vi "UT_006_LV to TOML.vi"() -> ()   [LabVIEW 2017]
uses:
  4ff207aa-191a-44af-8f7a-4e6e6b751422.vi
  <vilib>/addons/_JKI Toolkits/Caraya/classes/Assert/Assert True.vi
  lib/TOML to LabVIEW.vi
  <vilib>/addons/_JKI Toolkits/Caraya/classes/Assert/Assert Almost Equal_Float.vi
  <vilib>/addons/_JKI Toolkits/Caraya/classes/Test/Test.lvclass
  lib/TOML.lvlib
  <vilib>/addons/_JKI Toolkits/Caraya/classes/Assert/Assert.lvclass
panel:
  out "Cluster 2":T1={"2d-array-string"=[["a", "b", "c"], ["d", "e", "f"], ["g", "h", "i"]], "1d-array-float"=[3.14, nan, 1.123], "sub-cluster"={"string"="hello world", "path"=path "C:/dev/GitHub/.gitignore"}, "timestamp"=timestamp(3701448577.464638 s since 1904-01-01), "1d-array-cluster"=[{"string"="one", "int"=1}, {"string"="five", "int"=5}]}
  out "error out 2":errorcluster
  out "String":string
  in  "Cluster":T1={"2d-array-string"=[["a", "b", "c"], ["d", "e", "f"], ["g", "h", "i"]], "1d-array-float"=[3.14, nan, 1.123], "sub-cluster"={"string"="hello world", "path"=path "C:/dev/GitHub/.gitignore"}, "timestamp"=timestamp(3701448577.47 s since 1904-01-01), "1d-array-cluster"=[{"string"="one", "int"=1}, {"string"="five", "int"=5}]}
  out "error out":errorcluster
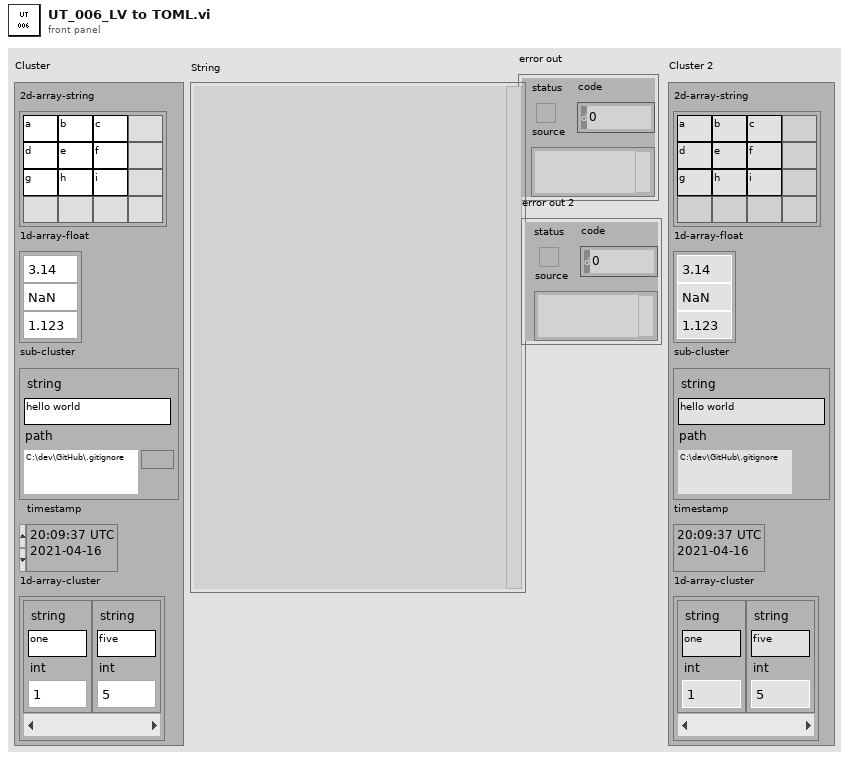
[diagram p1: front panel]
types:
  T1 = cluster{"2d-array-string":string[][], "1d-array-float":dbl[], "sub-cluster":cluster{"string":string, "path":path}, "timestamp":timestamp, "1d-array-cluster":cluster{"string":string, "int":i32}[]}
  T2 = typedef "TOML.lvlib/TOML Value.ctl" = cluster{"type":enum16{"Table", "Array", "String", "Integer", "Float", "Boolean", "Offset Date-Time", "Local Date-Time", "Local Date", "Local Time", "Path"}, "value":variant}
  T3 = cluster{"2d-array-string":bool[][], "1d-array-float":bool[], "sub-cluster":cluster{"string":bool, "path":bool}, "timestamp":bool, "1d-array-cluster":cluster{"string":bool, "int":bool}[]}
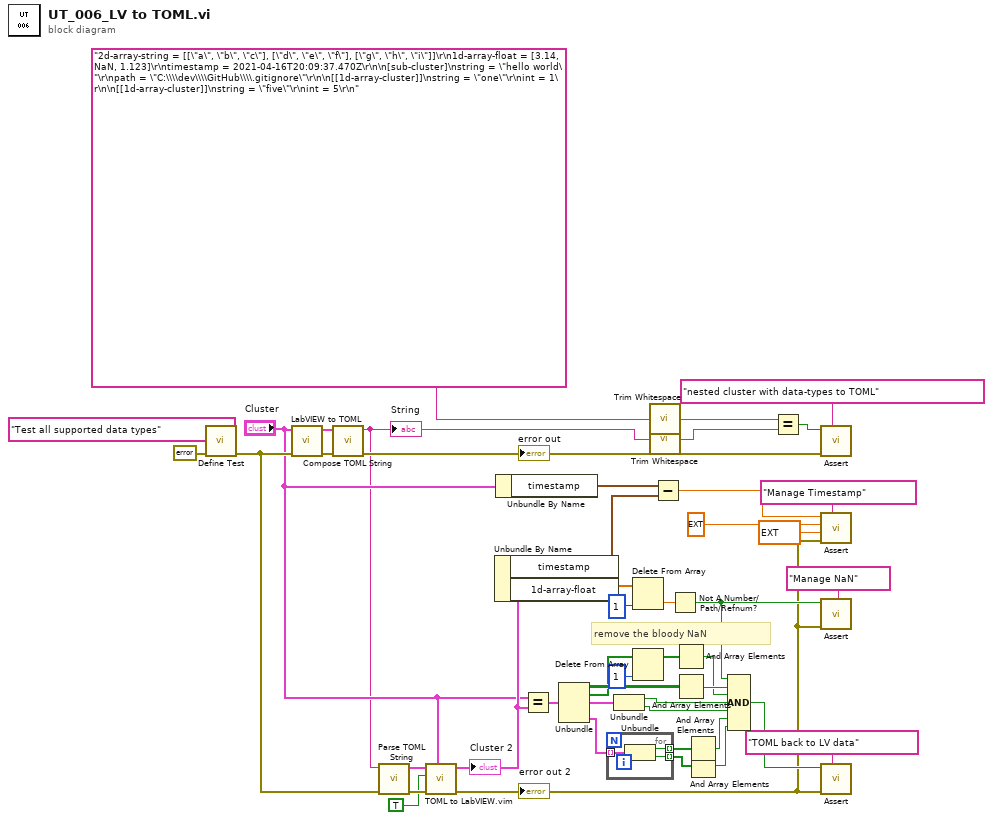
[diagram p0: block diagram]
diagram:
  # "remove the bloody NaN"
  n1 = call <vilib>:"Define Test.vi"("error in (no error)"=errorcluster {"status"=FALSE, "code"=0, "source"=""}, "Label (VI Title)"="Test all supported data types") -> ("error out"=w37:errorcluster)  [unwired: 9 in]
  n2 = call "LabVIEW to TOML.vi"("error in (no error)"=w37, "LV Value"="Cluster") -> ("error out"=w43:errorcluster, "TOML Value"=w36:T2)  [unwired: 7 in, 1 out]
  n3 = call "Compose TOML String.vi"("error in (no error)"=w43, "Value"=w36) -> ("error out"=w42:errorcluster, "String"=w2:string)  [unwired: 8 in]
  "error out" <- w42
  "String" <- w2
  n4 = call "Parse TOML String.vi"("error in (no error)"=w37, "String"=w2) -> ("error out"=w40:errorcluster, "Value"=w35:T2)  [unwired: 8 in]
  n5 = call "TOML to LabVIEW.vim"("datatype"="Cluster", "error in (no error)"=w40, "Error if missing element"=TRUE, "Value"=w35) -> ("error out"=w8:errorcluster, "LV Data"=w18:T1)  [unwired: 5 in, 1 out]
  "error out 2" <- w8
  "Cluster 2" <- w18
  n6 = Unbundle By Name(w18) -> ("timestamp"=w6:timestamp, "1d-array-float"=w17:dbl[])
  n7 = Unbundle By Name("Cluster") -> ("timestamp"=w12:timestamp)
  n8 = Equal?(x="Cluster", y=w18) -> (x = y?=w33:T3)
  n9 = Unbundle(w33) -> ("2d-array-string"=w28:bool[][], "1d-array-float"=w22:bool[], "sub-cluster"=w32:cluster{"string":bool, "path":bool}, "1d-array-cluster"=w31:cluster{"string":bool, "int":bool}[])  [unwired: 1 out]
  n10 = for {
    tunnel: w31 -> [w49] mode=indexing
    tunnel: [w48] -> w26 mode=indexing
    tunnel: [w47] -> w25 mode=indexing
    n11 = Unbundle(w49) -> ("string"=w48:bool, "int"=w47:bool)
  }
  n12 = Unbundle(w32) -> ("string"=w30:bool, "path"=w29:bool)
  n13 = Delete From Array(array=w17, index=1) -> (deleted portion=w15:dbl)  [unwired: 1 in, 1 out]
  n14 = Delete From Array(array=w22, index=1) -> (array with subset deleted=w20:bool[])  [unwired: 1 in, 1 out]
  n15 = call <vilib>:"Trim Whitespace.vi"("string"="2d-array-string = [[\"a\", \"b\", \"c\"], [\"d\", \"e\", \"f\"], [\"g\", \"h\", \"i\"]]\r\n1d-array-float = [3.14, NaN, 1.123]\r\ntimestamp = 2021-04-16T20:09:37.470Z\r\n\n[sub-cluster]\nstring = \"hello world\"\r\npath = \"C:\\\\dev\\\\GitHub\\\\.gitignore\"\r\n\n[[1d-array-cluster]]\nstring = \"one\"\r\nint = 1\r\n\n[[1d-array-cluster]]\nstring = \"five\"\r\nint = 5\r\n" ("x")) -> ("trimmed string"=w3:string)  [unwired: 1 in]
  n16 = call <vilib>:"Trim Whitespace.vi"("string"=w2) -> ("trimmed string"=w1:string)  [unwired: 1 in]
  n17 = Subtract(x=w12, y=w6) -> (x-y=w7:dbl)
  n18 = Not A Number/Path/Refnum?(number/path/refnum=w15) -> (NaN/Path/Refnum?=w10:bool)
  n19 = And Array Elements(Boolean array=w20) -> (logical AND=w19:bool)
  n20 = And Array Elements(Boolean array=w28) -> (logical AND=w27:bool)
  n21 = And Array Elements(Boolean array=w26) -> (logical AND=w24:bool)
  n22 = And Array Elements(Boolean array=w25) -> (logical AND=w23:bool)
  n23 = Compound Arithmetic op=AND(w10, w27, w19, w30, w29, w24, w23) -> (w14:bool)
  n24 = Equal?(x=w3, y=w1) -> (x = y?=w34:bool)
  n25 = call-poly <vilib>:"Assert.vi"("Label"="nested cluster with data-types to TOML" ("Label (VI Title)"), "error in (no error)"=w42, "True?"=w34) -> ()  [unwired: 8 in, 1 out]
  n26 = call-poly <vilib>:"Assert.vi"("Label"="Manage Timestamp" ("Label (VI Title)"), "error in (no error)"=w8, "Tolerance"=ext 0.00000100000000000000000004, "Y"=ext 0.0, "X"=w7) -> ()  [unwired: 6 in, 1 out]
  n27 = call-poly <vilib>:"Assert.vi"("Label"="Manage NaN" ("Label (VI Title)"), "error in (no error)"=w8, "True?"=w10) -> ()  [unwired: 8 in, 1 out]
  n28 = call-poly <vilib>:"Assert.vi"("Label"="TOML back to LV data" ("Label (VI Title)"), "error in (no error)"=w8, "True?"=w14) -> ()  [unwired: 8 in, 1 out]
